vi "predict_carriers.vi"(5 "Current/sensor index":i32 min=0 max=1 step=1, 6 "Modulation info":T1={"Fs full"=0.0, "Fs high"=0.0, "Fs low"=0.0, "Read size"=0, "FFT size low"=5000, "df low"=5000.0, "High carriers"=[], "Low carriers"=[], "Hi channels at low"=[7]} {"Hi channels at low" min=0 step=1; "Low carriers" format="%#_6p"; "High carriers" format="%#_6p"}, 7 "Low rate block start":bool, 8 "Low carrier amplitudes":cdb[](array[numeric]), 9 "KF in":T2 {"K" format="%#_2g"; "y lim" format="%#_3g"; "x lim" format="%#_2g"; "P" format="%#_2g"; "H" format="%#_3g"; "x" format="%#_3g"; "Q" format="%#_2g"; "R" format="%#_2g"; "B" format="%#_2g"; "A" format="%#_3g"}, 10 "Reset":bool, 11 "Config":T4={"IO params"={"Conversion"={"Rate"=4.0, "Num cards"=2, "Out channels"=4}, "Carriers"={"Phase shift"=180.0, "Levels"=[[0.8, 0.8, 0.8], [0.03, 0.03, 0.03]], "Delay samples"=73.15}, "TCP"={"Host"="192.168.1.15", "Port"=6666, "Buffering"=6, "Timeout"=6}, "Input channel sign"=[1, 1, 1]}, "High rate STFT"={"Win param"=101.5, "Window type"=61, "Win order"=2, "DFT size"=64, "Channels"=[7], "Oversample"=64}, "Low rate STFT"={"Win param"=120.0, "Window type"=61, "Win order"=8, "DFT size"=64, "Channels"=[7], "Oversample"=64}, "Filtering "=[]} {"Filtering"."Distortion"."Limit" format="%#_3p"; "Filtering"."Distortion"."LF cut" format="%#_3p"; "Filtering"."Kalman"."Measure noise" format="%#_3p"; "Filtering"."Kalman"."Process noise" format="%#_3p"; "Filtering"."Hum"."Limit" format="%#_3p"; "Filtering"."Hum"."Frequency" format="%#_4p"; "Low rate STFT"."Oversample" min=1 step=1; "Low rate STFT"."Channels" min=0 step=1; "Low rate STFT"."DFT size" min=1 step=1; "Low rate STFT"."Window type" items=["Rectangle"=0, "Hanning"=1, "Hamming"=2, "Blackman-Harris"=3, "Exact Blackman"=4, "Blackman"=5, "Flat Top"=6, "4 Term B-Harris "=7, "7 Term B-Harris"=8, "Low Sidelobe"=9, "Blackman Nuttall"=11, "Triangle"=30, "Bartlett-Hanning"=31, "Bohman"=32, "Parzen"=33, "Welch"=34, "Kaiser"=60, "Dolph-Chebyshev"=61, "Gaussian"=62]; "High rate STFT"."Oversample" min=1 step=1; "High rate STFT"."Channels" min=0 step=1; "High rate STFT"."DFT size" min=1 step=1; "High rate STFT"."Window type" items=["Rectangle"=0, "Hanning"=1, "Hamming"=2, "Blackman-Harris"=3, "Exact Blackman"=4, "Blackman"=5, "Flat Top"=6, "4 Term B-Harris "=7, "7 Term B-Harris"=8, "Low Sidelobe"=9, "Blackman Nuttall"=11, "Triangle"=30, "Bartlett-Hanning"=31, "Bohman"=32, "Parzen"=33, "Welch"=34, "Kaiser"=60, "Dolph-Chebyshev"=61, "Gaussian"=62]; "IO params"."Input channel sign" min=-1 max=1 step=1; "IO params"."Carriers"."Levels" min=0.0 step=0.1; "IO params"."Conversion"."Rate" format="%#_8g"}) -> (2 "KF out":T2 {"K" format="%#_2g"; "y lim" format="%#_3g"; "x lim" format="%#_2g"; "P" format="%#_2g"; "H" format="%#_3g"; "x" format="%#_3g"; "Q" format="%#_2g"; "R" format="%#_2g"; "B" format="%#_2g"; "A" format="%#_3g"}, 3 "Predicted carriers":dbl[](graph))   [LabVIEW 2026]
uses:
  utilities/kalman_filter.ctl
  <vilib>/Analysis/Matrix/Datatypes/RealMatrix.ctl
  ilemt_config.ctl
  system/IO_params.ctl
  stft_params.ctl
  <vilib>/Analysis/4window.llb/windowTd.ctl
  filter_params.ctl
  detrend_mode.ctl
  modulation_info.ctl
  <vilib>/Analysis/2dsp.llb/Inverse Real FFT.vi
  <vilib>/Analysis/Matrix/NI_Matrix.lvlib
  <vilib>/Analysis/NI_AALPro.lvlib
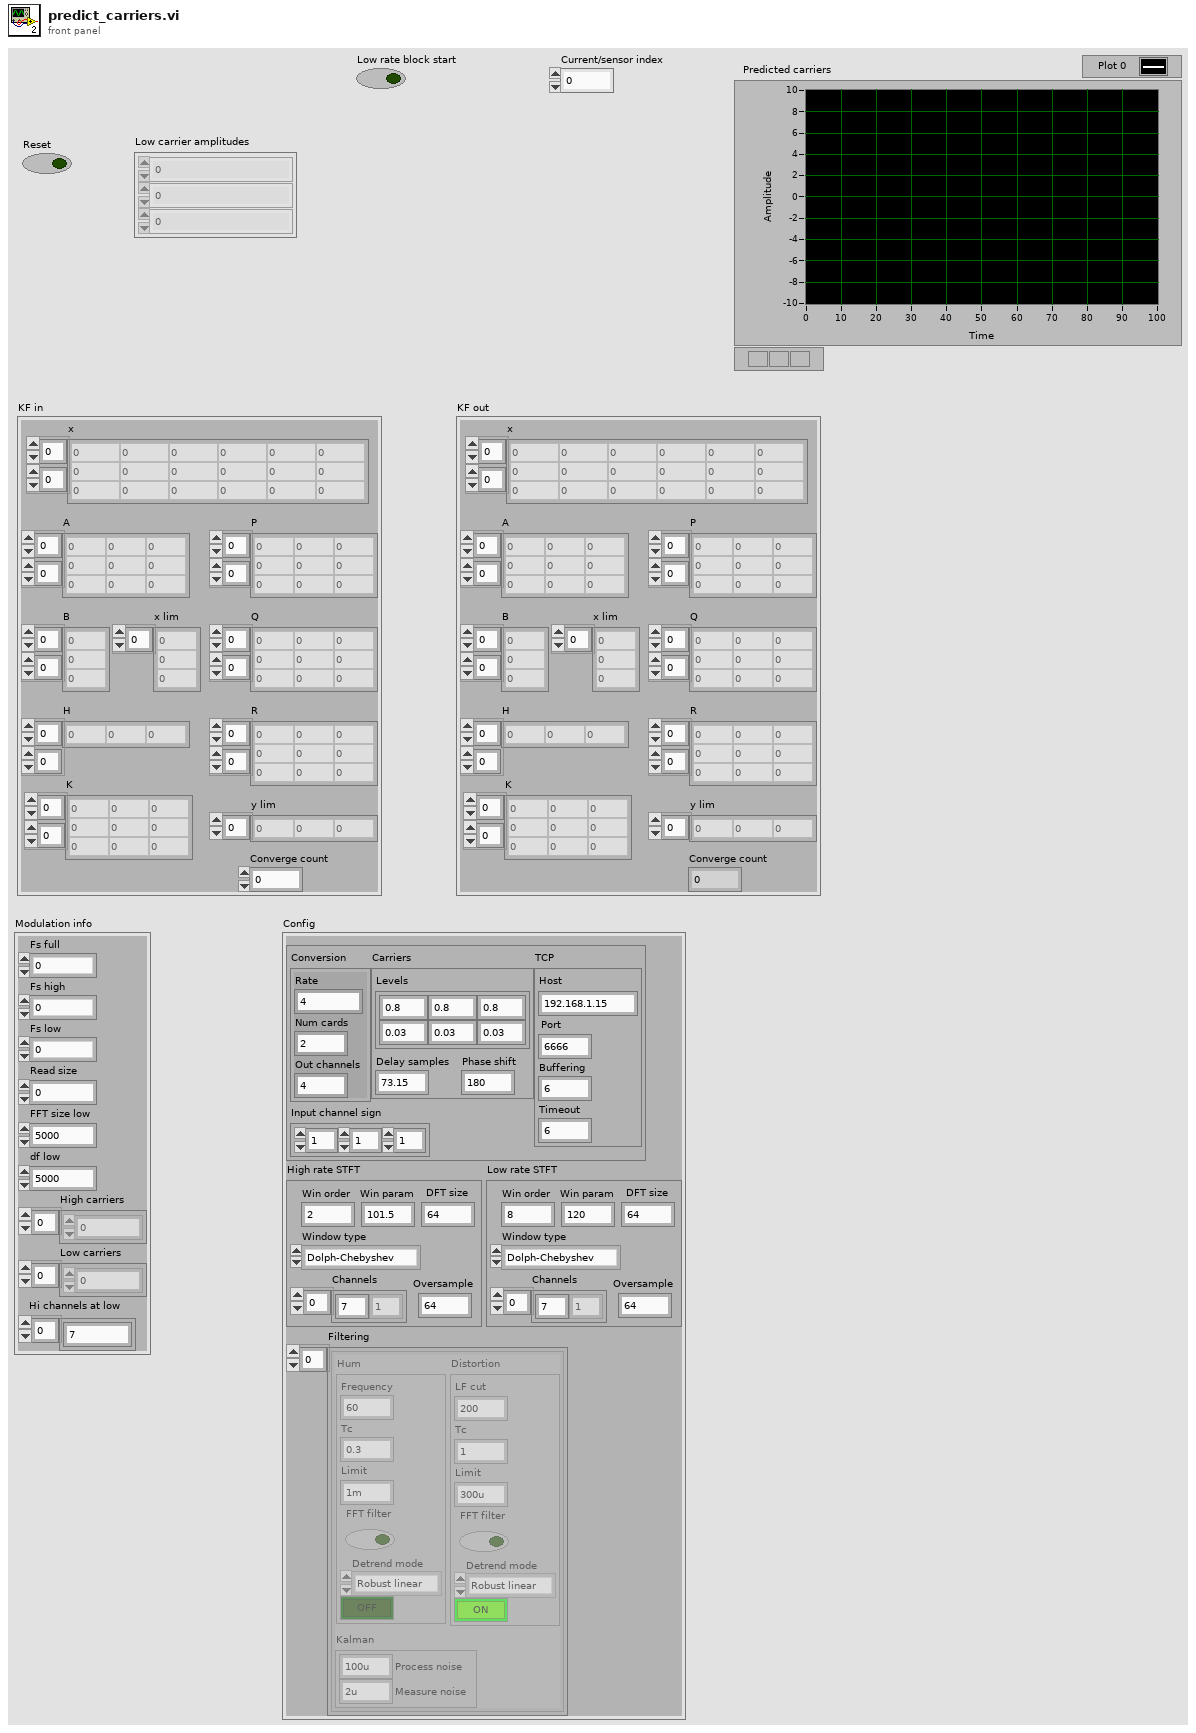
[diagram p1: front panel]
types:
  T1 = typedef "modulation_info.ctl" = cluster{"Fs full":dbl, "Fs high":dbl, "Fs low":dbl, "Read size":i32, "FFT size low":i32, "df low":dbl, "High carriers":dbl[], "Low carriers":dbl[], "Hi channels at low":i32[]}
  T2 = typedef "kalman_filter.ctl" = cluster{"A":T3, "B":T3, "H":T3, "Q":T3, "R":T3, "x":T3, "P":T3, "x lim":dbl[], "y lim":dbl[], "K":T3, "Converge count":i32}
  T3 = typedef "NI_Matrix.lvlib/RealMatrix.ctl" = dbl[][]
  T4 = typedef "ilemt_config.ctl" = cluster{"IO params":T5, "High rate STFT":T6, "Low rate STFT":T6, "Filtering ":T8[]}
  T5 = typedef "IO_params.ctl" = cluster{"Conversion":cluster{"Rate":dbl, "Num cards":u32, "Out channels":u32}, "Carriers":cluster{"Phase shift":dbl, "Levels":dbl[][], "Delay samples":dbl}, "TCP":cluster{"Host":string, "Port":i32, "Buffering":u32, "Timeout":u32}, "Input channel sign":i32[]}
  T6 = typedef "stft_params.ctl" = cluster{"Win param":dbl, "Window type":T7, "Win order":i32, "DFT size":i32, "Channels":i32[], "Oversample":i32}
  T7 = typedef "NI_AALPro.lvlib/windowTd.ctl" = u32
  T8 = typedef "filter_params.ctl" = cluster{"Hum":cluster{"Frequency":dbl, "Tc":dbl, "Limit":dbl, "FFT filter":bool, "Detrend mode":T9, "Enable":bool}, "Kalman":cluster{"Process noise":dbl, "Measure noise":dbl}, "Distortion":cluster{"LF cut":dbl, "Tc":dbl, "Limit":dbl, "FFT filter":bool, "Detrend mode":T9, "Enable":bool}}
  T9 = typedef "detrend_mode.ctl" = enum16{"Zero mean", "Linear", "Robust linear"}
  T10 = cluster{"Process noise":dbl, "Measure noise":dbl}
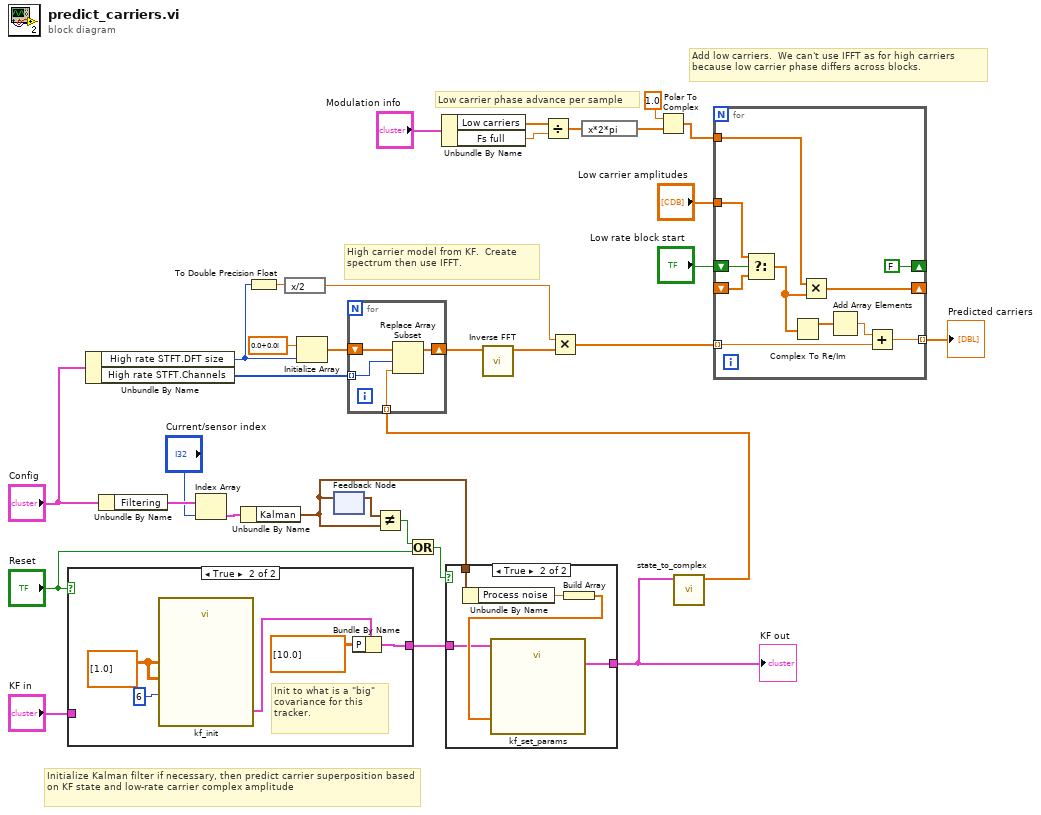
[diagram p0: block diagram]
diagram:
  # "Add low carriers.  We can't use IFFT as for high carriers because low carrier phase differs across blocks."
  # "High carrier model from KF.  Create spectrum then use IFFT."
  # "Initialize Kalman filter if necessary, then predict carrier superposition based on KF state and low-rate carrier complex amplitude"
  # "Low carrier phase advance per sample"
  n1 = case shown="True" "Reset" {
    tunnel: [w33 w34] -> w31
    tunnel: "KF in" -> [w33 _]
    frame False {
    }
    frame True {
      w37 = T3 [[1.0]] ("A")
      # "Init to what is a \"big\" covariance for this tracker."
      n2 = call "kf_init.vi"("A"=w37, "H"=w37, "x columns"=6) -> ("KF out"=w36:T2)  [unwired: 12 in]
      n3 = Bundle By Name(cluster=w36, "P"=T3 [[10.0]] ("A")) -> (w34:T2)
    }
  }
  n4 = Unbundle By Name("Config") -> ("High rate STFT.DFT size"=w9:i32, "High rate STFT.Channels"=w26:i32[])
  n5 = Unbundle By Name("Config") -> ("Filtering"=w5:T8[])
  n6 = Index Array(array=w5, index="Current/sensor index") -> (element=w2:T8)
  n7 = Unbundle By Name(w2) -> ("Kalman"=w1:T10)
  n8 = To Double Precision Float(number=w9) -> (double precision float=w15:dbl)
  n9 = expression code="x/2"(w15) -> (w13:dbl)
  n10 = Initialize Array(cdb 0.0+0.0i ("element"), w9) -> (w27:cdb[])
  n11 = feedback #1() -> (w30:T10)  [unwired: 1 in]
  n12 = feedback-in #1(w1) -> ()
  n13 = Not Equal?(x=w30, y=w1) -> (x != y?=w10:bool)
  n14 = Or(x=w10, y="Reset") -> (x .or. y?=w11:bool)
  n15 = Unbundle By Name("Modulation info") -> ("Low carriers"=w20:dbl[], "Fs full"=w19:dbl)
  n16 = case shown="True" w11 {
    tunnel: w31 -> [w39 w41]
    tunnel: w1 -> [_ w44]
    tunnel: [w39 w40] -> w32
    frame False {
    }
    frame True {
      n17 = Unbundle By Name(w44) -> ("Process noise"=w43:dbl)
      n18 = Build Array(w43) -> (w42:dbl[])
      n19 = call "kf_set_params.vi"("KF in"=w41, "Process noise"=w42) -> ("KF out"=w40:T2)  [unwired: 17 in]
    }
  }
  "KF out" <- w32
  n20 = Divide(x=w20, y=w19) -> (x/y=w18:dbl[])
  n21 = expression code="x*2*pi"(w18) -> (w17:dbl[])
  n22 = Polar To Complex(1:w17, 2:1.0 ("Fs full")) -> (0:w8:cdb[])
  n23 = call "state_to_complex.vi"("KF in"=w32) -> ("Amplitudes"=w25:cdb[])  [unwired: 10 in]
  n24 = for {
    tunnel: w26 -> [w46] mode=indexing
    tunnel: w25 -> [w47] mode=indexing
    shift-right: [w45] -> w24
    shift-left: w27 -> [w48]
    n25 = Replace Array Subset(array=w48, new element=w47, index=w46) -> (w45:cdb[])
  }
  n26 = call-poly <vilib>:"Inverse FFT.vi"("FFT {X}"=w24) -> ("X"=w14:dbl[])  [unwired: 9 in, 1 out]
  n27 = Multiply(x=w13, y=w14) -> (x*y=w7:dbl[])
  n28 = for {
    tunnel: w7 -> [w56] mode=indexing
    shift-right: [w55] -> _
    shift-left: _ -> [w57]
    tunnel: "Low carrier amplitudes" -> [w58]
    tunnel: w8 -> [w53]
    shift-right: [FALSE ("Low rate block start")] -> _
    shift-left: "Low rate block start" -> [w59]
    tunnel: [w49] -> w6 mode=indexing
    n29 = Select(t=w58, s=w59, f=w57) -> (s? t:f=w54:cdb[])
    n30 = Complex To Re/Im(x + iy=w54) -> (x=w51:dbl[])  [unwired: 1 out]
    n31 = Multiply(x=w53, y=w54) -> (x*y=w55:cdb[])
    n32 = Add Array Elements(numeric array=w51) -> (sum=w50:dbl)
    n33 = Add(x=w50, y=w56) -> (x+y=w49:dbl)
  }
  "Predicted carriers" <- w6
